vi "配置Bark参数.vi"(7 "FUN":enum16{"W", "R"}(ring), 11 "URLs":string[](array[string])) -> (3 "URLs 2":string[](array[string]))   [LabVIEW 2016]
uses:
  <vilib>/Utility/xml.llb/Write to XML File(string).vi
  <vilib>/Utility/xml.llb/Read From XML File(string).vi
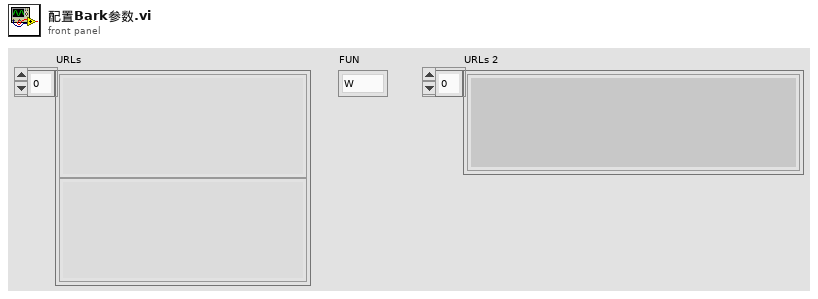
[diagram p1: front panel]
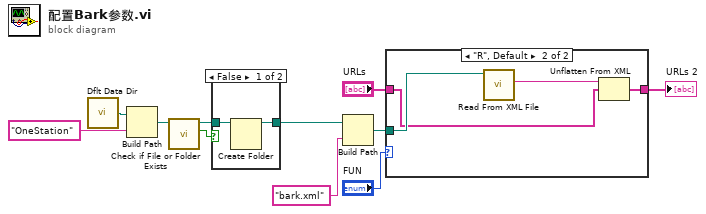
[diagram p0: block diagram]
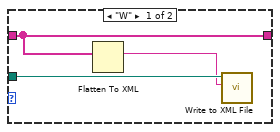
[diagram p3: hidden frame]
diagram:
  n1 = call <vilib>:"Dflt Data Dir.vi"() -> ("App:Default Data Directory"=w5:path)
  n2 = Build Path(base path=w5, name or relative path="OneStation" ("名称或相对路径")) -> (appended path=w4:path)
  n3 = call <vilib>:"Check if File or Folder Exists.vi"("path"=w4) -> ("file or folder exists?"=w3:bool, "dup path"=w2:path)  [unwired: 8 in, 1 out]
  n4 = case shown="False" w3 {
    tunnel: w2 -> [w13 w14]
    tunnel: [w12 w14] -> w1
    frame False {
      n5 = Create Folder(path (use dialog)=w13) -> (created path=w12:path)  [unwired: 2 in, 2 out]
    }
    frame True {
    }
  }
  n6 = Build Path(base path=w1, name or relative path="bark.xml" ("名称或相对路径")) -> (appended path=w9:path)
  n7 = case shown="\"R\", Default" "FUN" {
    tunnel: "URLs" -> [w15 w19]
    tunnel: w9 -> [w17 w21]
    tunnel: [w15 w18] -> w7
    frame "W" {
      n8 = Flatten To XML(anything=w15) -> (xml string=w16:string)
      n9 = call-poly <vilib>:"Write to XML File.vi"("XML Input"=w16, "XML File Path"=w17) -> ()  [unwired: 7 in, 3 out]
    }
    frame "R", Default {
      n10 = call-poly <vilib>:"Read From XML File.vi"("XML File Path"=w21) -> ("XML Elements"=w20:string)  [unwired: 8 in, 2 out]
      n11 = Unflatten From XML(xml string=w20, type=w19) -> (value=w18:string[])  [unwired: 1 in, 1 out]
    }
  }
  "URLs 2" <- w7
